vi "QuatToEuler.vi"(11 "RigidBodyOri":sgl[](array[numeric])) -> (3 "Array":sgl[](array[numeric]))   [LabVIEW 2013]
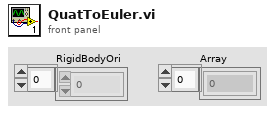
[diagram p1: front panel]
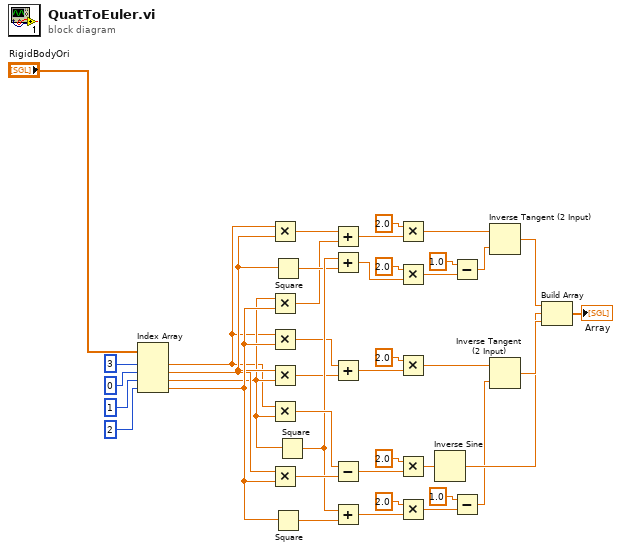
[diagram p0: block diagram]
diagram:
  n1 = Index Array(array="RigidBodyOri", index #1=3 ("index"), index #2=0 ("index"), index #3=1 ("index"), index #4=2 ("index")) -> (element #1=w30:sgl, element #2=w32:sgl, element #3=w31:sgl, element #4=w33:sgl)
  n2 = Multiply(x=w30, y=w32) -> (x*y=w2:sgl)
  n3 = Multiply(x=w31, y=w33) -> (x*y=w3:sgl)
  n4 = Multiply(x=w30, y=w33) -> (x*y=w27:sgl)
  n5 = Multiply(x=w32, y=w31) -> (x*y=w26:sgl)
  n6 = Multiply(x=w30, y=w31) -> (x*y=w34:sgl)
  n7 = Multiply(x=w32, y=w33) -> (x*y=w35:sgl)
  n8 = Square(x=w32) -> (x^2=w9:sgl)
  n9 = Square(x=w33) -> (x^2=w20:sgl)
  n10 = Square(x=w31) -> (x^2=w28:sgl)
  n11 = Add(x=w2, y=w3) -> (x+y=w4:sgl)
  n12 = Add(x=w28, y=w9) -> (x+y=w10:sgl)
  n13 = Add(x=w27, y=w26) -> (x+y=w25:sgl)
  n14 = Subtract(x=w34, y=w35) -> (x-y=w36:sgl)
  n15 = Add(x=w28, y=w20) -> (x+y=w19:sgl)
  n16 = Multiply(x=sgl 2.0, y=w4) -> (x*y=w6:sgl)
  n17 = Multiply(x=sgl 2.0, y=w10) -> (x*y=w8:sgl)
  n18 = Multiply(x=sgl 2.0, y=w25) -> (x*y=w23:sgl)
  n19 = Multiply(x=sgl 2.0, y=w36) -> (x*y=w37:sgl)
  n20 = Multiply(x=sgl 2.0, y=w19) -> (x*y=w21:sgl)
  n21 = Inverse Sine(1:w37) -> (0:w39:sgl)
  n22 = Subtract(x=sgl 1.0, y=w8) -> (x-y=w12:sgl)
  n23 = Subtract(x=sgl 1.0, y=w21) -> (x-y=w17:sgl)
  n24 = Inverse Tangent (2 Input)(1:w12, 2:w6) -> (0:w38:sgl)
  n25 = Inverse Tangent (2 Input)(1:w17, 2:w23) -> (0:w40:sgl)
  n26 = Build Array(w38, w39, w40) -> (→"Array":sgl[])
